vi "GetImageCollectionNumber2 (SubVI).vi"(8 "error in (no error)":errorcluster, 11 "Image in":T1) -> (0 "error out":errorcluster, 3 "Image #":i32)   [LabVIEW 2016]
uses:
  <vilib>/vision/Image Controls.llb/IMAQ Image.ctl
  <resource>/objmgr/IMAQImage.rc
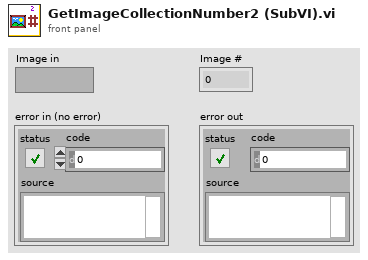
[diagram p1: front panel]
types:
  T1 = typedef "IMAQ Image.ctl" = refnum<image>
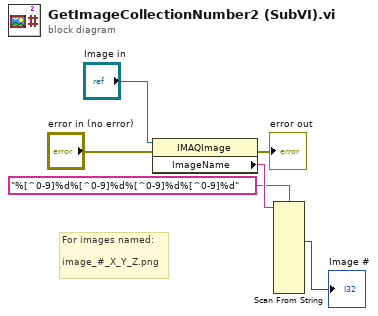
[diagram p0: block diagram]
diagram:
  # "For images named: \n\nimage_#_X_Y_Z.png"
  n1 = property class="IMAQImage"(reference="Image in", error in="error in (no error)") -> (error out=→"error out":errorcluster, "ImageName"=w3:string)  [unwired: 1 out]
  n2 = Scan From String(format string="%[^0-9]%d%[^0-9]%d%[^0-9]%d%[^0-9]%d", input string=w3) -> (output 2=→"Image #":i32)  [unwired: 17 in, 3 out]
